vi "FlatToRichnixnet_grpc_DbSetPropertyRequest.vi"(5 "OutputClusterType":T1, 11 "InputCluster":T3) -> (3 "OutputCluster":T1)   [LabVIEW 2025, in "grpc-xnet_client.lvlib"]
uses:
  nixnet_grpc_DbSetPropertyRequest_Flat.ctl
  nidevice_grpc_Session_Flat.ctl
  nixnet_grpc_DBProperty.ctl
  nixnet_grpc_U32Array_Flat.ctl
  nixnet_grpc_DbRefArray_Flat.ctl
  nixnet_grpc_DbSetPropertyRequest.ctl
  nixnet_grpc_DbSetPropertyRequest_dbproperty_id_enum/nixnet_grpc_DbSetPropertyRequest_dbproperty_id_enum.lvclass
  nixnet_grpc_DbSetPropertyRequest_property_value/nixnet_grpc_DbSetPropertyRequest_property_value.lvclass
  nidevice_grpc_Session.ctl
  grpc-xnet_client.lvlib
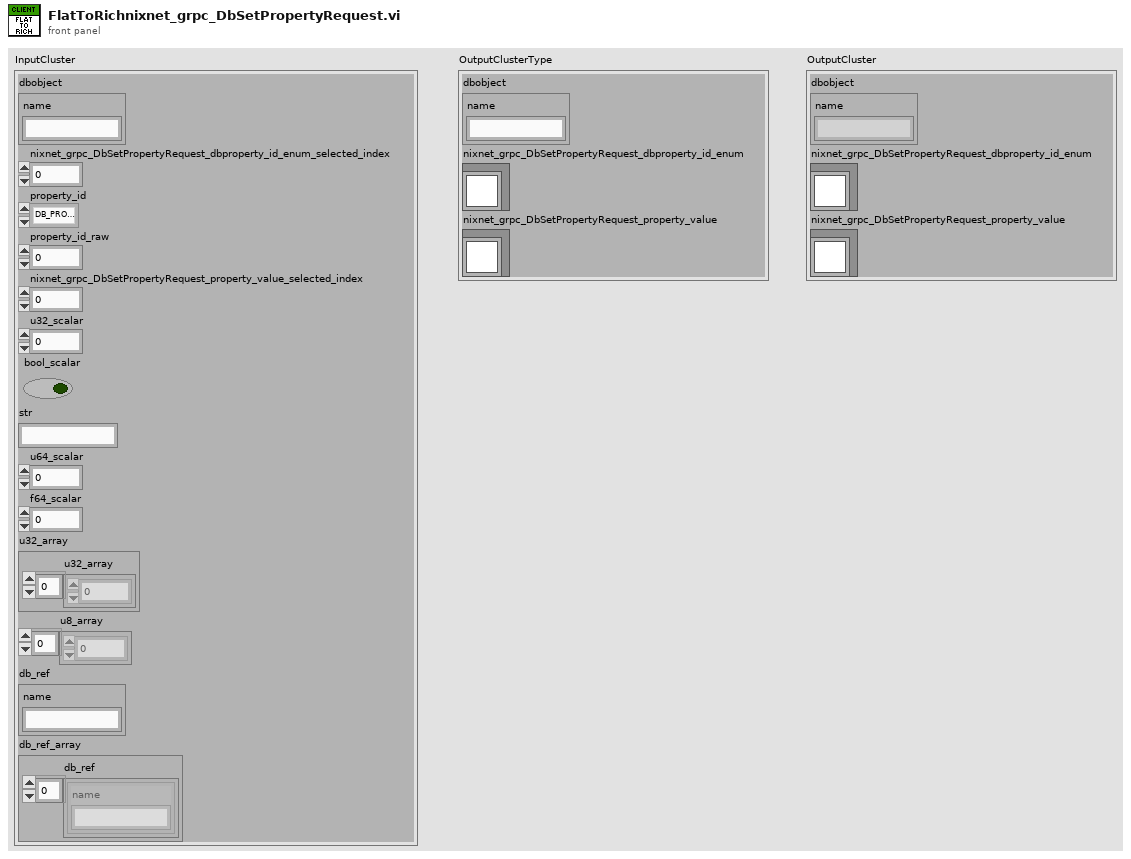
[diagram p1: front panel]
types:
  T1 = typedef "grpc-xnet_client.lvlib/nixnet_grpc_DbSetPropertyRequest.ctl" = cluster{"dbobject":T2, "nixnet_grpc_DbSetPropertyRequest_dbproperty_id_enum":refnum<class "nixnet_grpc_DbSetPropertyRequest_dbproperty_id_enum.lvclass">, "nixnet_grpc_DbSetPropertyRequest_property_value":refnum<class "nixnet_grpc_DbSetPropertyRequest_property_value.lvclass">}
  T2 = typedef "grpc-xnet_client.lvlib/nidevice_grpc_Session.ctl" = cluster{"name":string}
  T3 = typedef "grpc-xnet_client.lvlib/nixnet_grpc_DbSetPropertyRequest_Flat.ctl" = cluster{"dbobject":T4, "nixnet_grpc_DbSetPropertyRequest_dbproperty_id_enum_selected_index":i32, "property_id":T5, "property_id_raw":u32, "nixnet_grpc_DbSetPropertyRequest_property_value_selected_index":i32, "u32_scalar":u32, "bool_scalar":bool, "str":string, "u64_scalar":u64, "f64_scalar":dbl, "u32_array":T6, "u8_array":u8[], "db_ref":T4, "db_ref_array":T7}
  T4 = typedef "grpc-xnet_client.lvlib/nidevice_grpc_Session_Flat.ctl" = cluster{"name":string}
  T5 = typedef "grpc-xnet_client.lvlib/nixnet_grpc_DBProperty.ctl" = enum32{"DB_PROPERTY_UNSPECIFIED", "DB_PROPERTY_DATABASE_CLST_REFS", "DB_PROPERTY_DATABASE_NAME", "DB_PROPERTY_DATABASE_SHOW_INVALID_FROM_OPEN", "DB_PROPERTY_CLST_BAUD_RATE_64", "DB_PROPERTY_CLST_APPLICATION_PROTOCOL", "DB_PROPERTY_CLST_BAUD_RATE", "DB_PROPERTY_CLST_CAN_FD_BAUD_RATE_64", "DB_PROPERTY_CLST_CAN_FD_BAUD_RATE", "DB_PROPERTY_CLST_CAN_FD_ISO_MODE", "DB_PROPERTY_CLST_CAN_IO_MODE", "DB_PROPERTY_CLST_COMMENT", "DB_PROPERTY_CLST_CONFIG_STATUS", "DB_PROPERTY_CLST_DATABASE_REF", "DB_PROPERTY_CLST_ECU_REFS", "DB_PROPERTY_CLST_FLEX_RAY_ACT_PT_OFF", "DB_PROPERTY_CLST_FLEX_RAY_ALW_PASS_ACT", "DB_PROPERTY_CLST_FLEX_RAY_CAS_RX_L_MAX", "DB_PROPERTY_CLST_FLEX_RAY_CHANNELS", "DB_PROPERTY_CLST_FLEX_RAY_CLST_DRIFT_DMP", "DB_PROPERTY_CLST_FLEX_RAY_COLD_ST_ATS", "DB_PROPERTY_CLST_FLEX_RAY_CYCLE", "DB_PROPERTY_CLST_FLEX_RAY_DYN_SEG_START", "DB_PROPERTY_CLST_FLEX_RAY_DYN_SLOT_IDL_PH", "DB_PROPERTY_CLST_FLEX_RAY_LATEST_GUAR_DYN", "DB_PROPERTY_CLST_FLEX_RAY_LATEST_USABLE_DYN", "DB_PROPERTY_CLST_FLEX_RAY_LIS_NOISE", "DB_PROPERTY_CLST_FLEX_RAY_MACRO_PER_CYCLE", "DB_PROPERTY_CLST_FLEX_RAY_MACROTICK", "DB_PROPERTY_CLST_FLEX_RAY_MAX_WO_CLK_COR_FAT", "DB_PROPERTY_CLST_FLEX_RAY_MAX_WO_CLK_COR_PAS", "DB_PROPERTY_CLST_FLEX_RAY_MINISLOT", "DB_PROPERTY_CLST_FLEX_RAY_MINISLOT_ACT_PT", "DB_PROPERTY_CLST_FLEX_RAY_NIT", "DB_PROPERTY_CLST_FLEX_RAY_NIT_START", "DB_PROPERTY_CLST_FLEX_RAY_NM_VEC_LEN", "DB_PROPERTY_CLST_FLEX_RAY_NUM_MINISLT", "DB_PROPERTY_CLST_FLEX_RAY_NUM_STAT_SLT", "DB_PROPERTY_CLST_FLEX_RAY_OFF_COR_ST", "DB_PROPERTY_CLST_FLEX_RAY_PAYLD_LEN_DYN_MAX", "DB_PROPERTY_CLST_FLEX_RAY_PAYLD_LEN_MAX", "DB_PROPERTY_CLST_FLEX_RAY_PAYLD_LEN_ST", "DB_PROPERTY_CLST_FLEX_RAY_STAT_SLOT", "DB_PROPERTY_CLST_FLEX_RAY_SYM_WIN", "DB_PROPERTY_CLST_FLEX_RAY_SYM_WIN_START", "DB_PROPERTY_CLST_FLEX_RAY_SYNC_NODE_MAX", "DB_PROPERTY_CLST_FLEX_RAY_TSS_TX", "DB_PROPERTY_CLST_FLEX_RAY_USE_WAKEUP", "DB_PROPERTY_CLST_FLEX_RAY_WAKE_SYM_RX_IDL", "DB_PROPERTY_CLST_FLEX_RAY_WAKE_SYM_RX_LOW", "DB_PROPERTY_CLST_FLEX_RAY_WAKE_SYM_RX_WIN", "DB_PROPERTY_CLST_FLEX_RAY_WAKE_SYM_TX_IDL", "DB_PROPERTY_CLST_FLEX_RAY_WAKE_SYM_TX_LOW", "DB_PROPERTY_CLST_FRM_REFS", "DB_PROPERTY_CLST_LIN_SCHEDULES", "DB_PROPERTY_CLST_LIN_TICK", "DB_PROPERTY_CLST_NAME", "DB_PROPERTY_CLST_PDU_REFS", "DB_PROPERTY_CLST_PD_US_REQD", "DB_PROPERTY_CLST_PROTOCOL", "DB_PROPERTY_CLST_SIG_REFS", "DB_PROPERTY_FRM_APPLICATION_PROTOCOL", "DB_PROPERTY_FRM_CAN_EXT_ID", "DB_PROPERTY_FRM_CAN_IO_MODE", "DB_PROPERTY_FRM_CAN_TIMING_TYPE", "DB_PROPERTY_FRM_CAN_TX_TIME", "DB_PROPERTY_FRM_CLUSTER_REF", "DB_PROPERTY_FRM_COMMENT", "DB_PROPERTY_FRM_CONFIG_STATUS", "DB_PROPERTY_FRM_DEFAULT_PAYLOAD", "DB_PROPERTY_FRM_FLEX_RAY_BASE_CYCLE", "DB_PROPERTY_FRM_FLEX_RAY_CH_ASSIGN", "DB_PROPERTY_FRM_FLEX_RAY_CYCLE_REP", "DB_PROPERTY_FRM_FLEX_RAY_IN_CYC_REP_CH_ASSIGNS", "DB_PROPERTY_FRM_FLEX_RAY_IN_CYC_REP_ENABLED", "DB_PROPERTY_FRM_FLEX_RAY_IN_CYC_REP_IDS", "DB_PROPERTY_FRM_FLEX_RAY_PREAMBLE", "DB_PROPERTY_FRM_FLEX_RAY_STARTUP", "DB_PROPERTY_FRM_FLEX_RAY_SYNC", "DB_PROPERTY_FRM_FLEX_RAY_TIMING_TYPE", "DB_PROPERTY_FRM_ID", "DB_PROPERTY_FRM_LIN_CHECKSUM", "DB_PROPERTY_FRM_MUX_DATA_MUX_SIG_REF", "DB_PROPERTY_FRM_MUX_IS_MUXED", "DB_PROPERTY_FRM_MUX_STATIC_SIG_REFS", "DB_PROPERTY_FRM_MUX_SUBFRAME_REFS", "DB_PROPERTY_FRM_NAME", "DB_PROPERTY_FRM_PDU_START_BITS", "DB_PROPERTY_FRM_PDU_UPDATE_BITS", "DB_PROPERTY_FRM_PDU_REFS", "DB_PROPERTY_FRM_PAYLOAD_LEN", "DB_PROPERTY_FRM_SIG_REFS", "DB_PROPERTY_FRM_VARIABLE_PAYLOAD", "DB_PROPERTY_SIG_BYTE_ORDR", "DB_PROPERTY_SIG_COMMENT", "DB_PROPERTY_SIG_CONFIG_STATUS", "DB_PROPERTY_SIG_DATA_TYPE", "DB_PROPERTY_SIG_DEFAULT", "DB_PROPERTY_SIG_FRAME_REF", "DB_PROPERTY_SIG_MAX", "DB_PROPERTY_SIG_MIN", "DB_PROPERTY_SIG_MUX_IS_DATA_MUX", "DB_PROPERTY_SIG_MUX_IS_DYNAMIC", "DB_PROPERTY_SIG_MUX_VALUE", "DB_PROPERTY_SIG_MUX_SUBFRM_REF", "DB_PROPERTY_SIG_NAME", "DB_PROPERTY_SIG_NAME_UNIQUE_TO_CLUSTER", "DB_PROPERTY_SIG_NUM_BITS", "DB_PROPERTY_SIG_PDU_REF", "DB_PROPERTY_SIG_SCALE_FAC", "DB_PROPERTY_SIG_SCALE_OFF", "DB_PROPERTY_SIG_START_BIT", "DB_PROPERTY_SIG_UNIT", "DB_PROPERTY_SUBFRM_CONFIG_STATUS", "DB_PROPERTY_SUBFRM_DYN_SIG_REFS", "DB_PROPERTY_SUBFRM_FRM_REF", "DB_PROPERTY_SUBFRM_MUX_VALUE", "DB_PROPERTY_SUBFRM_NAME", "DB_PROPERTY_SUBFRM_NAME_UNIQUE_TO_CLUSTER", "DB_PROPERTY_SUBFRM_PDU_REF", "DB_PROPERTY_ECU_CLST_REF", "DB_PROPERTY_ECU_COMMENT", "DB_PROPERTY_ECU_CONFIG_STATUS", "DB_PROPERTY_ECU_FLEX_RAY_IS_COLDSTART", "DB_PROPERTY_ECU_FLEX_RAY_CONNECTED_CHS", "DB_PROPERTY_ECU_FLEX_RAY_STARTUP_FRAME_REF", "DB_PROPERTY_ECU_FLEX_RAY_WAKEUP_CHS", "DB_PROPERTY_ECU_FLEX_RAY_WAKEUP_PTRN", "DB_PROPERTY_ECU_RX_FRM_REFS", "DB_PROPERTY_ECU_TX_FRM_REFS", "DB_PROPERTY_ECU_LIN_CONFIG_NAD", "DB_PROPERTY_ECU_LIN_FUNCTION_ID", "DB_PROPERTY_ECU_LIN_INITIAL_NAD", "DB_PROPERTY_ECU_LIN_MASTER", "DB_PROPERTY_ECU_LINP2MIN", "DB_PROPERTY_ECU_LIN_PROTOCOL_VER", "DB_PROPERTY_ECU_LINS_TMIN", "DB_PROPERTY_ECU_LIN_SUPPLIER_ID", "DB_PROPERTY_ECU_NAME", "DB_PROPERTY_ECU_J1939_NODE_NAME", "DB_PROPERTY_ECU_J1939_PREFERRED_ADDRESS", "DB_PROPERTY_LIN_SCHED_CLST_REF", "DB_PROPERTY_LIN_SCHED_COMMENT", "DB_PROPERTY_LIN_SCHED_CONFIG_STATUS", "DB_PROPERTY_LIN_SCHED_ENTRIES", "DB_PROPERTY_LIN_SCHED_NAME", "DB_PROPERTY_LIN_SCHED_PRIORITY", "DB_PROPERTY_LIN_SCHED_RUN_MODE", "DB_PROPERTY_LIN_SCHED_ENTRY_COLLISION_RES_SCHED", "DB_PROPERTY_LIN_SCHED_ENTRY_DELAY", "DB_PROPERTY_LIN_SCHED_ENTRY_EVENT_ID", "DB_PROPERTY_LIN_SCHED_ENTRY_FRAMES", "DB_PROPERTY_LIN_SCHED_ENTRY_NAME", "DB_PROPERTY_LIN_SCHED_ENTRY_NAME_UNIQUE_TO_CLUSTER", "DB_PROPERTY_LIN_SCHED_ENTRY_NC_FF_DATA_BYTES", "DB_PROPERTY_LIN_SCHED_ENTRY_SCHED", "DB_PROPERTY_LIN_SCHED_ENTRY_TYPE", "DB_PROPERTY_PDU_CLUSTER_REF", "DB_PROPERTY_PDU_COMMENT", "DB_PROPERTY_PDU_CONFIG_STATUS", "DB_PROPERTY_PDU_DEFAULT_PAYLOAD", "DB_PROPERTY_PDU_FRM_REFS", "DB_PROPERTY_PDU_MUX_DATA_MUX_SIG_REF", "DB_PROPERTY_PDU_MUX_IS_MUXED", "DB_PROPERTY_PDU_MUX_STATIC_SIG_REFS", "DB_PROPERTY_PDU_MUX_SUBFRAME_REFS", "DB_PROPERTY_PDU_NAME", "DB_PROPERTY_PDU_PAYLOAD_LEN", "DB_PROPERTY_PDU_SIG_REFS"}
  T6 = typedef "grpc-xnet_client.lvlib/nixnet_grpc_U32Array_Flat.ctl" = cluster{"u32_array":u32[]}
  T7 = typedef "grpc-xnet_client.lvlib/nixnet_grpc_DbRefArray_Flat.ctl" = cluster{"db_ref":T4[]}
  T8 = typedef "grpc-xnet_client.lvlib/nixnet_grpc_U32Array.ctl" = cluster{"u32_array":u32[]}
  T9 = typedef "grpc-xnet_client.lvlib/nixnet_grpc_DbRefArray.ctl" = cluster{"db_ref":T2[]}
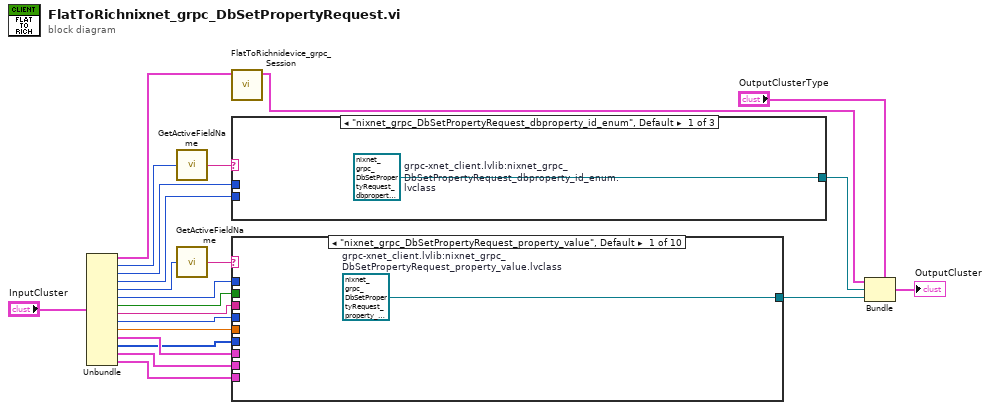
[diagram p0: block diagram]
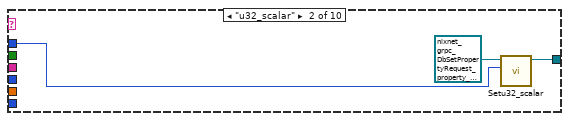
[diagram p2: hidden frame]
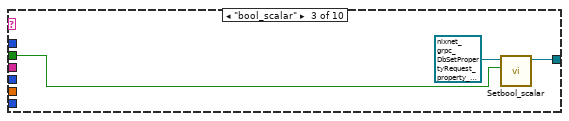
[diagram p3: hidden frame]
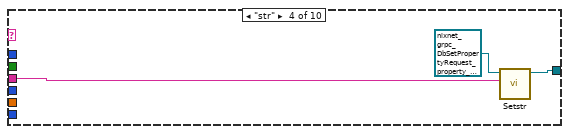
[diagram p4: hidden frame]
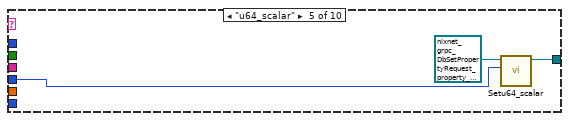
[diagram p5: hidden frame]
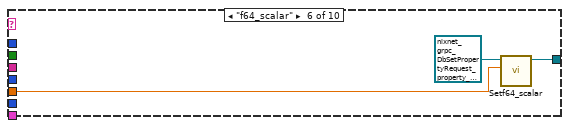
[diagram p6: hidden frame]
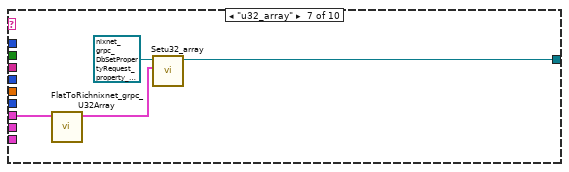
[diagram p7: hidden frame]
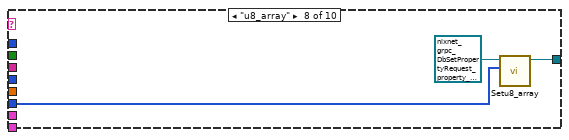
[diagram p8: hidden frame]
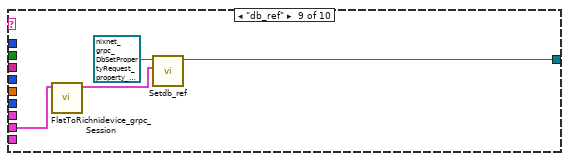
[diagram p9: hidden frame]
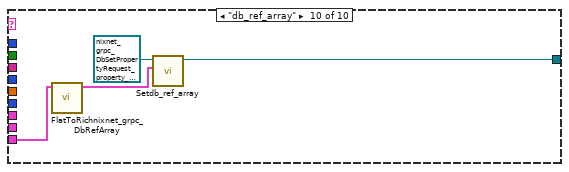
[diagram p10: hidden frame]
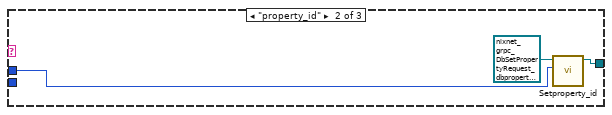
[diagram p11: hidden frame]
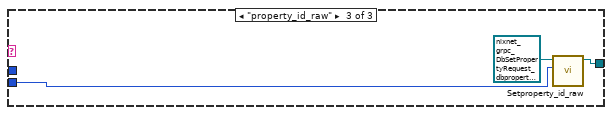
[diagram p12: hidden frame]
diagram:
  n1 = Unbundle "Unbundle"("InputCluster") -> ("dbobject"=w19:T4, "nixnet_grpc_DbSetPropertyRequest_dbproperty_id_enum_selected_index"=w17:i32, "property_id"=w14:T5, "property_id_raw"=w13:u32, "nixnet_grpc_DbSetPropertyRequest_property_value_selected_index"=w12:i32, "u32_scalar"=w9:u32, "bool_scalar"=w8:bool, "str"=w7:string, "u64_scalar"=w6:u64, "f64_scalar"=w5:dbl, "u32_array"=w4:T6, "u8_array"=w3:u8[], "db_ref"=w2:T4, "db_ref_array"=w1:T7)
  n2 = call "GetActiveFieldName.vi"("protobuf index"=w17) -> ("oneof field name"=w16:string)
  n3 = call "GetActiveFieldName.vi"("protobuf index"=w12) -> ("oneof field name"=w11:string)
  n4 = call "FlatToRichnidevice_grpc_Session.vi"("InputCluster"=w19) -> ("OutputCluster"=w18:T2)  [unwired: 10 in]
  n5 = case "nixnet_grpc_DbSetPropertyRequest_dbproperty_id_enum" shown="\"nixnet_grpc_DbSetPropertyRequest_dbproperty_id_enum\", Default" w16 {
    tunnel: [w23 w25 w28] -> w15
    tunnel: w14 -> [_ w26 _]
    tunnel: w13 -> [_ _ w29]
    frame "nixnet_grpc_DbSetPropertyRequest_dbproperty_id_enum", Default {
      w23 = refnum<class "nixnet_grpc_DbSetPropertyRequest_dbproperty_id_enum.lvclass"> refnum  # grpc-xnet_client.lvlib:nixnet_grpc_DbSetPropertyRequest_dbproperty_id_enum.lvclass
    }
    frame "property_id" {
      n6 = call "Setproperty_id.vi"("Set_Val"=w26, "OneOfTemplate in"=refnum<class "nixnet_grpc_DbSetPropertyRequest_dbproperty_id_enum.lvclass"> refnum) -> ("OneOfTemplate out"=w25:refnum<class "nixnet_grpc_DbSetPropertyRequest_dbproperty_id_enum.lvclass">)  [unwired: 8 in, 1 out]
    }
    frame "property_id_raw" {
      n7 = call "Setproperty_id_raw.vi"("Set_Val"=w29, "OneOfTemplate in"=refnum<class "nixnet_grpc_DbSetPropertyRequest_dbproperty_id_enum.lvclass"> refnum) -> ("OneOfTemplate out"=w28:refnum<class "nixnet_grpc_DbSetPropertyRequest_dbproperty_id_enum.lvclass">)  [unwired: 8 in, 1 out]
    }
  }
  n8 = case "nixnet_grpc_DbSetPropertyRequest_property_value" shown="\"nixnet_grpc_DbSetPropertyRequest_property_value\", Default" w11 {
    tunnel: [w30 w32 w35 w38 w41 w44 w47 w51 w54 w58] -> w10
    tunnel: w9 -> [_ w33 _ _ _ _ _ _ _ _]
    tunnel: w8 -> [_ _ w36 _ _ _ _ _ _ _]
    tunnel: w7 -> [_ _ _ w39 _ _ _ _ _ _]
    tunnel: w6 -> [_ _ _ _ w42 _ _ _ _ _]
    tunnel: w5 -> [_ _ _ _ _ w45 _ _ _ _]
    tunnel: w4 -> [_ _ _ _ _ _ w49 _ _ _]
    tunnel: w3 -> [_ _ _ _ _ _ _ w52 _ _]
    tunnel: w2 -> [_ _ _ _ _ _ _ _ w56 _]
    tunnel: w1 -> [_ _ _ _ _ _ _ _ _ w60]
    frame "nixnet_grpc_DbSetPropertyRequest_property_value", Default {
      w30 = refnum<class "nixnet_grpc_DbSetPropertyRequest_property_value.lvclass"> refnum  # grpc-xnet_client.lvlib:nixnet_grpc_DbSetPropertyRequest_property_value.lvclass
    }
    frame "u32_scalar" {
      n9 = call "Setu32_scalar.vi"("Set_Val"=w33, "OneOfTemplate in"=refnum<class "nixnet_grpc_DbSetPropertyRequest_property_value.lvclass"> refnum) -> ("OneOfTemplate out"=w32:refnum<class "nixnet_grpc_DbSetPropertyRequest_property_value.lvclass">)  [unwired: 8 in, 1 out]
    }
    frame "bool_scalar" {
      n10 = call "Setbool_scalar.vi"("Set_Val"=w36, "OneOfTemplate in"=refnum<class "nixnet_grpc_DbSetPropertyRequest_property_value.lvclass"> refnum) -> ("OneOfTemplate out"=w35:refnum<class "nixnet_grpc_DbSetPropertyRequest_property_value.lvclass">)  [unwired: 8 in, 1 out]
    }
    frame "str" {
      n11 = call "Setstr.vi"("Set_Val"=w39, "OneOfTemplate in"=refnum<class "nixnet_grpc_DbSetPropertyRequest_property_value.lvclass"> refnum) -> ("OneOfTemplate out"=w38:refnum<class "nixnet_grpc_DbSetPropertyRequest_property_value.lvclass">)  [unwired: 8 in, 1 out]
    }
    frame "u64_scalar" {
      n12 = call "Setu64_scalar.vi"("Set_Val"=w42, "OneOfTemplate in"=refnum<class "nixnet_grpc_DbSetPropertyRequest_property_value.lvclass"> refnum) -> ("OneOfTemplate out"=w41:refnum<class "nixnet_grpc_DbSetPropertyRequest_property_value.lvclass">)  [unwired: 8 in, 1 out]
    }
    frame "f64_scalar" {
      n13 = call "Setf64_scalar.vi"("Set_Val"=w45, "OneOfTemplate in"=refnum<class "nixnet_grpc_DbSetPropertyRequest_property_value.lvclass"> refnum) -> ("OneOfTemplate out"=w44:refnum<class "nixnet_grpc_DbSetPropertyRequest_property_value.lvclass">)  [unwired: 8 in, 1 out]
    }
    frame "u32_array" {
      n14 = call "FlatToRichnixnet_grpc_U32Array.vi"("InputCluster"=w49) -> ("OutputCluster"=w48:T8)  [unwired: 10 in]
      n15 = call "Setu32_array.vi"("Set_Val"=w48, "OneOfTemplate in"=refnum<class "nixnet_grpc_DbSetPropertyRequest_property_value.lvclass"> refnum) -> ("OneOfTemplate out"=w47:refnum<class "nixnet_grpc_DbSetPropertyRequest_property_value.lvclass">)  [unwired: 8 in, 1 out]
    }
    frame "u8_array" {
      n16 = call "Setu8_array.vi"("Set_Val"=w52, "OneOfTemplate in"=refnum<class "nixnet_grpc_DbSetPropertyRequest_property_value.lvclass"> refnum) -> ("OneOfTemplate out"=w51:refnum<class "nixnet_grpc_DbSetPropertyRequest_property_value.lvclass">)  [unwired: 8 in, 1 out]
    }
    frame "db_ref" {
      n17 = call "FlatToRichnidevice_grpc_Session.vi"("InputCluster"=w56) -> ("OutputCluster"=w55:T2)  [unwired: 10 in]
      n18 = call "Setdb_ref.vi"("Set_Val"=w55, "OneOfTemplate in"=refnum<class "nixnet_grpc_DbSetPropertyRequest_property_value.lvclass"> refnum) -> ("OneOfTemplate out"=w54:refnum<class "nixnet_grpc_DbSetPropertyRequest_property_value.lvclass">)  [unwired: 8 in, 1 out]
    }
    frame "db_ref_array" {
      n19 = call "FlatToRichnixnet_grpc_DbRefArray.vi"("InputCluster"=w60) -> ("OutputCluster"=w59:T9)  [unwired: 10 in]
      n20 = call "Setdb_ref_array.vi"("Set_Val"=w59, "OneOfTemplate in"=refnum<class "nixnet_grpc_DbSetPropertyRequest_property_value.lvclass"> refnum) -> ("OneOfTemplate out"=w58:refnum<class "nixnet_grpc_DbSetPropertyRequest_property_value.lvclass">)  [unwired: 8 in, 1 out]
    }
  }
  n21 = Bundle "Bundle"(cluster="OutputClusterType", "dbobject"=w18, "nixnet_grpc_DbSetPropertyRequest_dbproperty_id_enum"=w15, "nixnet_grpc_DbSetPropertyRequest_property_value"=w10) -> (→"OutputCluster":T1)
